vi "Self Alias.vi"(11 "Base Event in":refnum<class "Base Event.lvclass">) -> (2 "Self Alias":string, 3 "Base Event out":refnum<class "Base Event.lvclass">)   [LabVIEW 2021, in "jettl.lvlib" / "Base Event.lvlib" / "Base Event.lvclass"]
uses:
  Base Event.lvclass
  Base Event.lvclass/Base Event.ctl
  Addresses/Addresses/Addresses.lvclass
  C:/git/jettl/jettl/jettl/jettl/jettl.lvclass
  C:/git/jettl/jettl/Merge Error Msg Strategy/Merge Error/Merge Error.lvclass
  C:/git/jettl/jettl/jettl/Event/Event.lvclass
  C:/git/jettl/jettl/Create Msg Strategy/Create/Create.lvclass
  C:/git/jettl/jettl/jettl/Last Ack Created Msg Strategy/Last Ack Created/Last Ack Created.lvclass
  C:/git/jettl/jettl/jettl/Last Ack Creator Msg Strategy/Last Ack Creator/Last Ack Creator.lvclass
  C:/git/jettl/jettl/Override Error Msg Strategy/Override Error/Override Error.lvclass
  C:/git/jettl/jettl/Setup Msg Strategy/Setup/Setup.lvclass
  C:/git/jettl/jettl/Teardown Msg Strategy/Teardown/Teardown.lvclass
  C:/git/jettl/jettl/jettl/Base Event/Base Event/Base Event.lvclass
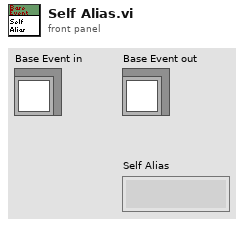
[diagram p1: front panel]
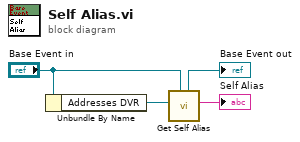
[diagram p0: block diagram]
diagram:
  n1 = Unbundle By Name("Base Event in") -> ("Addresses DVR"=w3:refnum<data-value>)
  n2 = call "Get Self Alias.vi"("jettl in"="Base Event in", "Addresses DVR"=w3) -> ("Self Alias"=→"Self Alias":string, "jettl out"=→"Base Event out":refnum<class "Base Event.lvclass">)  [unwired: 8 in]
